vi "Read Measurement 2 Channels.vi"(6 "Measurement Type (0: Phase)":i32(ring) items=["Phase", "Delay", "DelayRR", "DelayRF", "DelayFR", "DelayFF"], 8 "error in (no error)":errorcluster, 9 "Channel 2 (2: Channel 2)":i32(ring)=2 items=["Channel 1"=1, "Channel 2"=2, "Channel 3"=3, "Channel 4"=4], 10 "Channel 1 (1: Channel 1)":i32(ring)=1 items=["Channel 1"=1, "Channel 2"=2, "Channel 3"=3, "Channel 4"=4], 11 "EDU-X-1002A in":refnum<class "EDU-X-1002A.lvclass">) -> (0 "error out":errorcluster, 1 "Measurement":dbl, 2 "Units":string, 3 "EDU-X-1002A out":refnum<class "EDU-X-1002A.lvclass">)   [LabVIEW 2020, in "Controlador.lvlib" / "EDU-X-1002A.lvclass"]
uses:
  EDU-X-1002A.lvclass
  C:/Users/scrap/Fork/Modulo_Cloneable_DQMH/Libraries/Controlador/Class/Osciloscope/Osciloscope.lvclass
  Osciloscope/Osciloscope.lvclass/Osciloscope.ctl
  Osciloscope/Read COM.vi
  <instrlib>/Agilent 2000 3000 X-Series/Public/Data/Read Measurement (Current Value).vi
  Osciloscope/Osciloscope.lvclass
  <instrlib>/Agilent 2000 3000 X-Series/Agilent 2000 3000 X-Series.lvlib
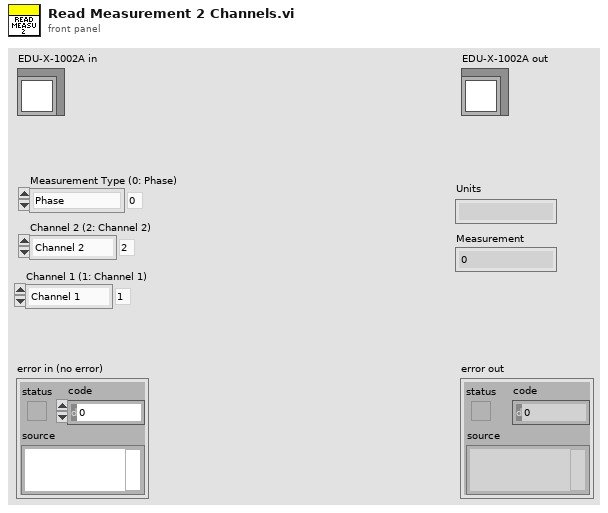
[diagram p1: front panel]
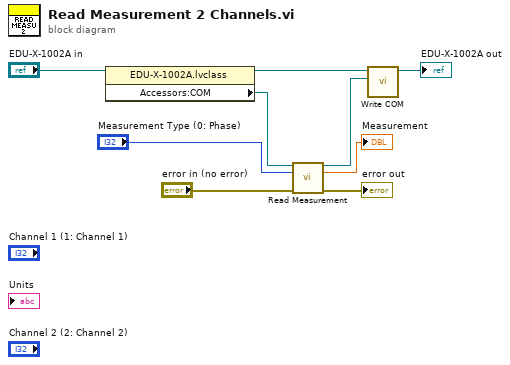
[diagram p0: block diagram]
diagram:
  n1 = property class="EDU-X-1002A.lvclass"(reference="EDU-X-1002A in") -> (reference out=w9:refnum<class "EDU-X-1002A.lvclass">, "Accessors:COM"=w6:refnum<visa-resource-name>)  [unwired: 1 in, 1 out]
  n2 = call-poly <instrlib>:"Read Measurement.vi"("VISA resource name"=w6, "Measurement Type (0: Peak-Peak)"="Measurement Type (0: Phase)", "error in (no error)"="error in (no error)") -> ("VISA resource name out"=w5:refnum<visa-resource-name>, "Result Value"=→"Measurement":dbl, "error out"=→"error out":errorcluster)  [unwired: 10 in]
  n3 = call "Write COM.vi"("COM"=w5, "Osciloscope in"=w9) -> ("Osciloscope out"=→"EDU-X-1002A out":refnum<class "EDU-X-1002A.lvclass">)  [unwired: 8 in, 1 out]
